vi "Starter Kit 2.0 Custom FPGA Main.vi"() -> ()   [LabVIEW 2011]
doc: "This VI implements the low level control of the motors and sensor for the Starter Kit 2.0 robot. The functionality of this VI is similar to the fixed FPGA personality used by the Starter Kit API."
uses:
  <vilib>/Platform/TimedLoop/XDataNode/timing_clust.ctl
  <vilib>/Platform/TimedLoop/XDataNode/nitl_modes.ctl
  <vilib>/Platform/TimedLoop/XDataNode/wakeup.ctl
  <vilib>/robotics/Utilities/Encoder Count Encoding.ctl
  Support VIs/Starter Kit 2.0 FPGA Globals.vi
  <vilib>/robotics/Utilities/FPGA Utilities/Count Two Phase Digital Encoder.vi
  <vilib>/rvi/eio/common/nirviEmuTemplateMethod_errors.vi
  <vilib>/robotics/Utilities/FPGA Utilities/Generate Digital Pulse (uSec).vi
  <vilib>/Platform/TimedLoop/XDataNode/XDataNode.xnode
  <vilib>/eio/EIONode/EIONode.xnode
  <vilib>/addons/control/pid/fpga.llb/XNode/niFpgaPID.xnode
  <vilib>/Platform/TimedLoop/XDataNode/XDNodeRunTimeDep.lvlib
  <vilib>/robotics/Utilities/NI_Robotics Utilities.lvlib
  <vilib>/robotics/Utilities/FPGA Utilities/NI_Robotics_FPGA Utilities.lvlib
  <instrlib>/Parallax PING)))/FPGA/NI_Robotics_Parallax PING))) (FPGA).lvlib
  <instrlib>/Hitec HS400 Series/FPGA/NI_Robotics_Hitec HS400 Series (FPGA).lvlib
  <instrlib>/Devantech CMPS03/FPGA/NI_Robotics_Devantech CMPS03 (FPGA).lvlib
panel:
  out "right counts":i32
  out "left counts":i32
  out "CMPS03 angle":fxp<+,20,16>
  out "CMPS 03 timed out":bool
  in  "FPGA LED":bool
  in  "ModB/AO0":fxp<+/-,20,5> format="%.17g"
  in  "ModB/AO1":fxp<+/-,20,5> format="%.17g"
  out "ModA/AI0":fxp<+/-,26,5> format="%.23g"
  out "ModA/AI1":fxp<+/-,26,5> format="%.23g"
  in  "Port7/DIO0_PWM":T1={"period (us)"=20000, "pulse width (us)"=1500}
  in  "Port7/DIO1_PWM":T1={"period (us)"=20000, "pulse width (us)"=1500}
  in  "Port3/DIO1":bool
  in  "Port3/DIO1_write":bool
  in  "Port3/DIO0":bool
  in  "Port3/DIO0_write":bool
  in  "hs400_0_ccw offset":fxp<+/-,32,4>
  in  "hs400_0_ccw angle":fxp<+/-,32,4>
  out "PING)))_0_timeout":bool
  out "PING)))_0_dist":fxp<+,32,8> format="%.27g"
  out "DCmotor_1_ccw vel":fxp<+/-,32,11>
  out "DCmotor_0_ccw vel":fxp<+/-,32,11>
  in  "DCmotor_1_ccw vel sp":fxp<+/-,32,11>
  in  "DCmotor_0_ccw vel sp":fxp<+/-,32,11>
  in  "stop":bool
  in  "motor PID gains":T2={"proportional gain (Kc)"=0.25, "integral gain (Kc*Ts/Ti)"=0.08984375, "derivative gain (Kc*Td/Ts)"=0.01171875}
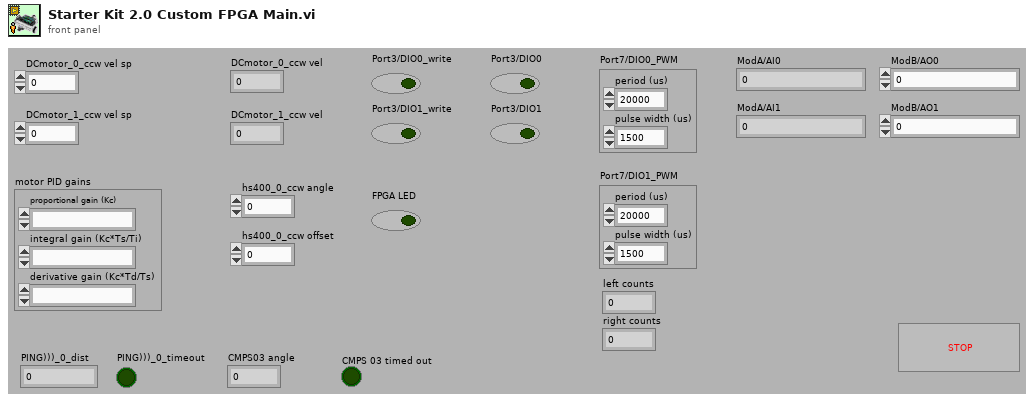
[diagram p1: front panel]
types:
  T1 = cluster{"period (us)":u32, "pulse width (us)":u32}
  T2 = cluster{"proportional gain (Kc)":fxp<+/-,16,8>, "integral gain (Kc*Ts/Ti)":fxp<+/-,16,8>, "derivative gain (Kc*Td/Ts)":fxp<+/-,16,8>}
  T3 = cluster{"PID gains":cluster{"proportional gain (Kc)":fxp<+/-,16,8>, "integral gain (Kc*Ts/Ti)":fxp<+/-,16,8>, "derivative gain (Kc*Td/Ts)":fxp<+/-,16,8>}, "output range":cluster{"output high":fxp<+/-,16,16>, "output low":fxp<+/-,16,16>}, "setpoint":fxp<+/-,16,16>, "channel index":u16}
  T4 = cluster{"PID gains (x 2^8)":cluster{"proportional gain (Kc)":i16, "integral gain (Kc*Ts/Ti)":i16, "derivative gain (Kc*Td/Ts)":i16}, "output range":cluster{"output high":i16, "output low":i16}, "setpoint":i16, "channel index":u16}
  T5 = typedef "XDNodeRunTimeDep.lvlib/timing_clust.ctl" = cluster{"Expected End [f-1]":u64, "Actual End [f-1]":u64, "Finished Late? [f-1]":bool, "Expected End [i-1]":u64, "Actual End [i-1]":u64, "Finished Late? [i-1]":bool, "Expected Start [i]":u64, "Actual Start [i]":u64, "Expected Start [f]":u64, "Actual Start [f]":u64, "Source Name":string, "Structure Name":string, "Period":i64, "Deadline":i64, "Offset":i64, "Start":i64, "Priority":i32, "Timeout":i32, "Mode":T6, "Wakeup Reason":T7, "Error":errorcluster, "Source Type":string, "Secondary Source Type":string, "Global End Time":u64, "Global Start Time":u64, "Frame Duration":u64, "Iteration Duration":u64, "Assigned CPU":i32, "I/O Scan Engine Mode":u32}
  T6 = typedef "XDNodeRunTimeDep.lvlib/nitl_modes.ctl" = enum32{"No Change", "Process missed periods, maintain original phase", "Discard missed periods, maintain original phase", "Process missed periods, ignore original phase", "Discard missed periods, ignore original phase"}
  T7 = typedef "XDNodeRunTimeDep.lvlib/wakeup.ctl" = enum32{"Normal", "Aborted", "Asynchronous wakeup", "Timing source error", "Timed loop error", "Timeout"}
  T8 = typedef "NI_Robotics Utilities.lvlib/Encoder Count Encoding.ctl" = enum16{"X1", "X2", "X4"}
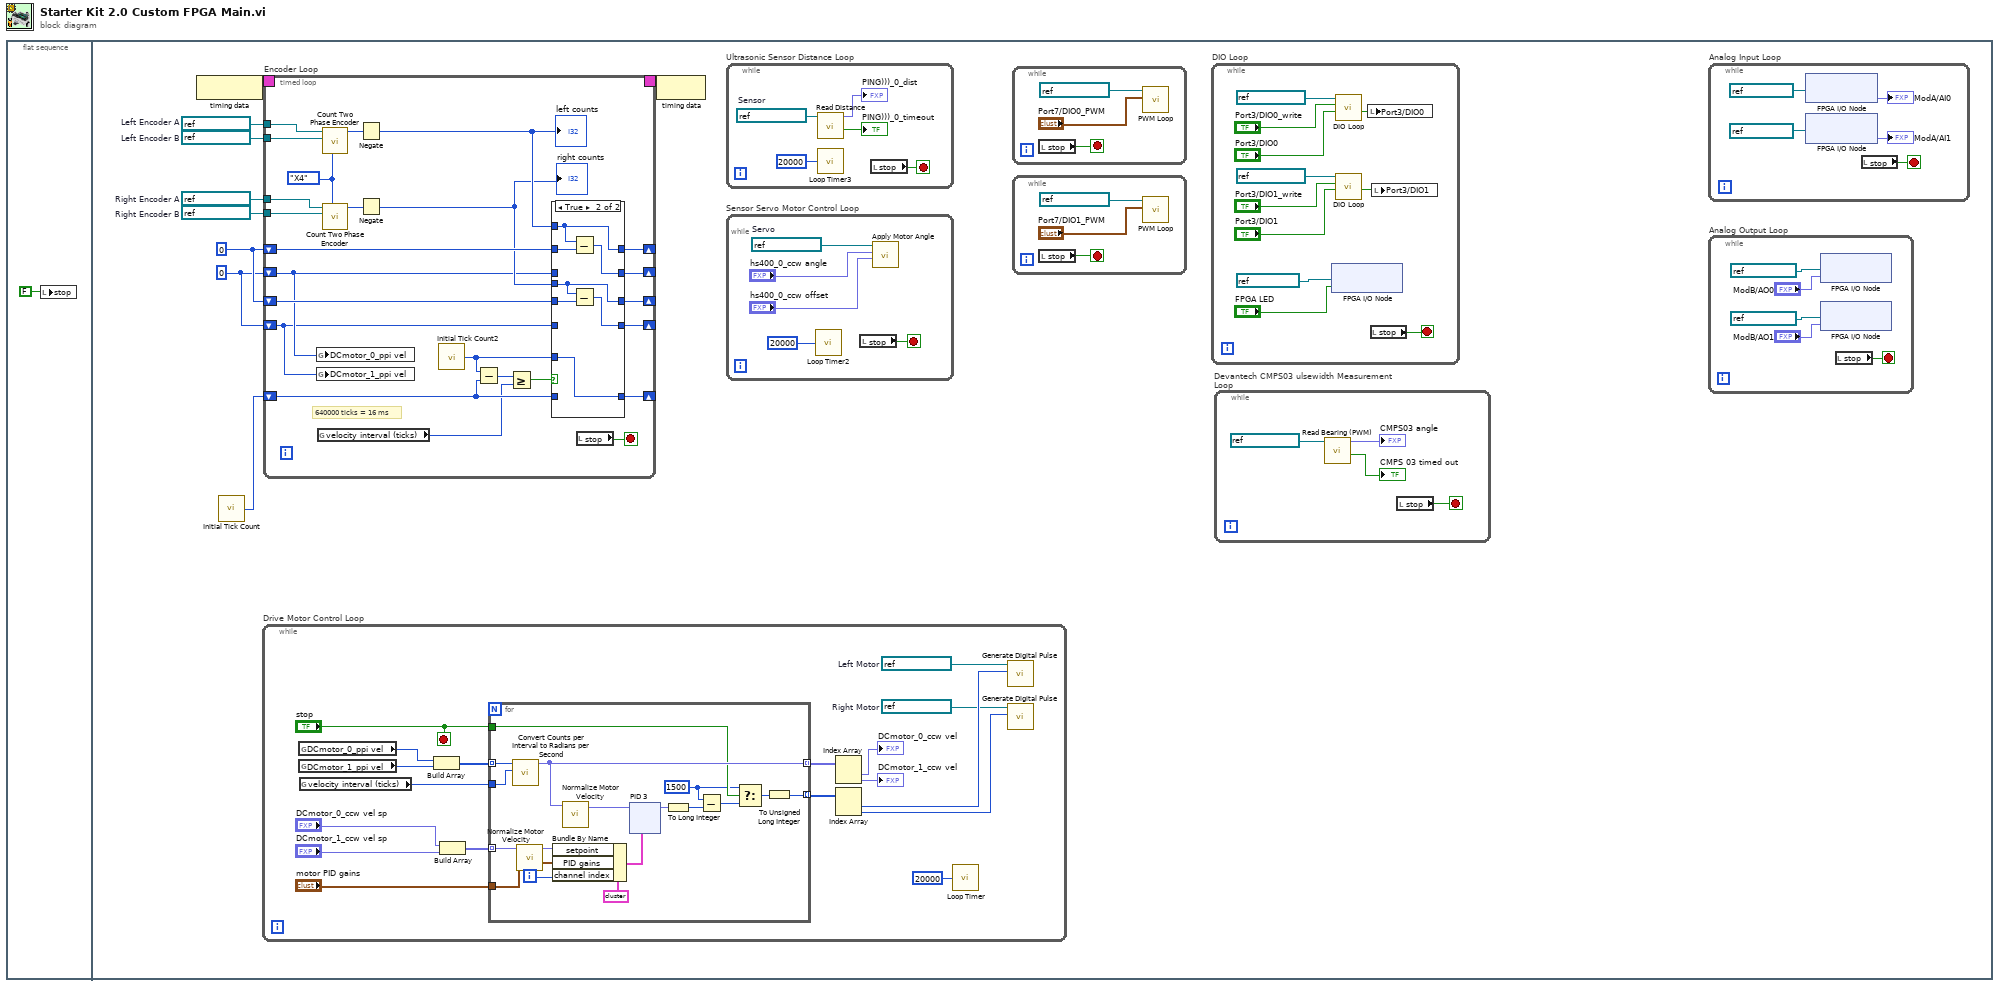
[diagram p0: block diagram]
diagram:
  n1 = flat-sequence {
    frame #0 {
      n2 = local write "stop"(FALSE ("stop")) -> ()
    }
    frame #1 {
      w2 = refnum<k21> "Port0/DIO3"  # Right Encoder B
      w3 = refnum<k21> "Port0/DIO2"  # Right Encoder A
      w4 = refnum<k21> "Port0/DIO1"  # Left Encoder B
      w5 = refnum<k21> "Port0/DIO0"  # Left Encoder A
      w6 = 0
      w7 = 0 ("Reset Position Value")
      n3 = node-c288() -> (w10:T5)
      n4 = call "Initial Tick Count"() -> ("Tick Count(Ticks)"=w8:u32)
      n5 = while "Drive Motor Control Loop" {
        stop <- "stop" stop-if-true
        w48 = refnum<k21> "Port0/DIO5"  # Right Motor
        w49 = refnum<k21> "Port0/DIO4"  # Left Motor
        n6 = global read "Starter Kit 2.0 FPGA Globals.vi" "DCmotor_0_ppi vel"() -> (w43:i32)
        n7 = global read "Starter Kit 2.0 FPGA Globals.vi" "DCmotor_1_ppi vel"() -> (w42:i32)
        n8 = global read "Starter Kit 2.0 FPGA Globals.vi" "velocity interval (ticks)"() -> (w44:u32)
        n9 = Build Array(w43, w42) -> (w57:i32[])
        n10 = Build Array("DCmotor_0_ccw vel sp", "DCmotor_1_ccw vel sp") -> (w55:fxp<+/-,32,11>[])
        n11 = for {
          tunnel: "motor PID gains" -> [w73]
          tunnel: w57 -> [w72] mode=indexing
          tunnel: w44 -> [w71]
          tunnel: [w70] -> w56 mode=indexing
          tunnel: w55 -> [w60] mode=indexing
          tunnel: "stop" -> [w64]
          tunnel: [w66] -> w54 mode=indexing
          i -> [w74]
          w63 = 1500 ("y")
          n12 = call "Convert Counts per Interval to Radians per Second.vi"("interval (ticks)"=w71, "velocity (pulses/interval)"=w72) -> ("velocity (rad/s)"=w70:fxp<+/-,32,11>)  [unwired: 9 in]
          n13 = call "Normalize Motor Velocity.vi"("velocity (rad/s)"=w60) -> ("normalized velocity"=w67:fxp<+/-,16,16>)  [unwired: 10 in]
          n14 = Bundle By Name(cluster=T3 {"PID gains"={"proportional gain (Kc)"=0.00390625, "integral gain (Kc*Ts/Ti)"=0.00390625, "derivative gain (Kc*Td/Ts)"=0.00390625}, "output range"={"output high"=500.0, "output low"=-500.0}, "setpoint"=0.0, "channel index"=0} ("configuration"), "setpoint"=w67, "PID gains"=w73, "channel index"=w74) -> (w75:T3)
          n15 = call "Normalize Motor Velocity.vi"("velocity (rad/s)"=w70) -> ("normalized velocity"=w69:fxp<+/-,16,16>)  [unwired: 10 in]
          n16 = xnode ("PID 3")("process variable"=w69, "configuration"=w75) -> ("output"=w68:fxp<+/-,16,16>)  [unwired: 1 in, 1 out]
          n17 = To Long Integer(number=w68) -> (32bit integer=w65:i32)
          n18 = Subtract(x=w63, y=w65) -> (x-y=w62:i32)
          n19 = Select(t=w63, s=w64, f=w62) -> (s? t:f=w61:i32)
          n20 = To Unsigned Long Integer(number=w61) -> (unsigned 32bit integer=w66:u32)
        }
        n21 = Index Array(array=w56) -> (element #1=→"DCmotor_0_ccw vel":fxp<+/-,32,11>, element #2=→"DCmotor_1_ccw vel":fxp<+/-,32,11>)  [unwired: 2 in]
        n22 = Index Array(array=w54) -> (element #1=w53:u32, element #2=w50:u32)  [unwired: 2 in]
        n23 = call "Loop Timer"("Count(uSec)"=u32 20000) -> ()  [unwired: 1 out]
        n24 = call-poly <vilib>:"Generate Digital Pulse.vi"("pulse width (uSec)"=w53, "FPGA digital output"=w49) -> ()  [unwired: 10 in]
        n25 = call-poly <vilib>:"Generate Digital Pulse.vi"("pulse width (uSec)"=w50, "FPGA digital output"=w48) -> ()  [unwired: 10 in]
      }
      n26 = timed-loop "Encoder Loop" {
        timing: w10 -> [_]
        timing-out: [_] -> w9
        shift-right: [w130] -> _
        shift-left: w8 -> [w135]
        shift-right: [w131] -> _
        shift-left: w7 -> [w133]
        shift-right: [w132] -> _
        shift-left: w6 -> [w116]
        shift-right: [w128] -> _
        shift-left: w7 -> [w129]
        shift-right: [w127] -> _
        shift-left: w6 -> [w115]
        tunnel: w5 -> [w123]
        tunnel: w4 -> [w122]
        tunnel: w3 -> [w120]
        tunnel: w2 -> [w119]
        stop <- w124 stop-if-true
        w117 = Encoder_Count_Encoding."X4" ("count multiplier (X1)")
        # "640000 ticks = 16 ms"
        n27 = global write "Starter Kit 2.0 FPGA Globals.vi" "DCmotor_0_ppi vel"(w116) -> ()
        n28 = global write "Starter Kit 2.0 FPGA Globals.vi" "DCmotor_1_ppi vel"(w115) -> ()
        n29 = global read "Starter Kit 2.0 FPGA Globals.vi" "velocity interval (ticks)"() -> (w114:u32)
        n30 = call-poly <vilib>:"Count Two Phase Encoder.vi"("count encoding (X1)"=w117, "phase B FPGA digital input"=w122, "phase A FPGA digital input"=w123) -> ("new count"=w121:i32)  [unwired: 7 in, 1 out]
        n31 = call-poly <vilib>:"Count Two Phase Encoder.vi"("count encoding (X1)"=w117, "phase B FPGA digital input"=w119, "phase A FPGA digital input"=w120) -> ("new count"=w118:i32)  [unwired: 7 in, 1 out]
        n32 = Negate(x=w121) -> (-x=w126:i32)
        "left counts" <- w126
        n33 = Negate(x=w118) -> (-x=w125:i32)
        "right counts" <- w125
        n34 = call "Initial Tick Count2"() -> ("Tick Count(Ticks)"=w134:u32)
        n35 = Subtract(x=w134, y=w135) -> (x-y=w137:u32)
        n36 = Greater Or Equal?(x=w137, y=w114) -> (x >= y?=w136:bool)
        n37 = case shown="True" w136 {
          tunnel: w134 -> [_ w148]
          tunnel: w135 -> [w142 _]
          tunnel: [w142 w148] -> w130
          tunnel: w133 -> [w141 w149]
          tunnel: [w141 w147] -> w131
          tunnel: w126 -> [_ w147]
          tunnel: [w140 w146] -> w132
          tunnel: w116 -> [w140 _]
          tunnel: w129 -> [w139 w145]
          tunnel: w115 -> [w138 _]
          tunnel: [w139 w144] -> w128
          tunnel: [w138 w143] -> w127
          tunnel: w125 -> [_ w144]
          frame False {
          }
          frame True {
            n38 = Subtract(x=w147, y=w149) -> (x-y=w146:i32)
            n39 = Subtract(x=w144, y=w145) -> (x-y=w143:i32)
          }
        }
        n40 = local read "stop"() -> (w124:bool)
      }
      n41 = node-c288(w9) -> ()
      n42 = while "Ultrasonic Sensor Distance Loop" {
        stop <- w112 stop-if-true
        w109 = refnum<k21> "Port0/DIO6"  # Sensor
        n43 = call <instrlib>:"Read Distance.vi"("trigger/echo line"=w109) -> ("timed out?"=→"PING)))_0_timeout":bool, "distance (m)"=→"PING)))_0_dist":fxp<+,32,8>)  [unwired: 9 in]
        n44 = call "Loop Timer3"("Count(uSec)"=u32 20000 ("sensor period (15000 us)")) -> ()  [unwired: 1 out]
        n45 = local read "stop"() -> (w112:bool)
      }
      n46 = while "Sensor Servo Motor Control Loop" {
        stop <- w108 stop-if-true
        w107 = refnum<k21> "Port0/DIO7"  # Servo
        n47 = call "Loop Timer2"("Count(uSec)"=u32 20000) -> ()  [unwired: 1 out]
        n48 = local read "stop"() -> (w108:bool)
        n49 = call <instrlib>:"Apply Motor Angle.vi"("ccw angle offset (rad)"="hs400_0_ccw offset", "ccw angle (rad)"="hs400_0_ccw angle", "digital output line"=w107) -> ()  [unwired: 9 in]
      }
      n50 = while {
        stop <- w41 stop-if-true
        n51 = local read "stop"() -> (w41:bool)
        n52 = call "PWM Loop.vi"("PWM"="Port7/DIO0_PWM", "FPGA I/O"=refnum<k21> "Port7/DIO0" ("FPGA I/O In")) -> ()  [unwired: 10 in]
      }
      n53 = while {
        stop <- w38 stop-if-true
        n54 = local read "stop"() -> (w38:bool)
        n55 = call "PWM Loop.vi"("PWM"="Port7/DIO1_PWM", "FPGA I/O"=refnum<k21> "Port7/DIO1" ("FPGA I/O In")) -> ()  [unwired: 10 in]
      }
      n56 = while "DIO Loop" {
        stop <- w27 stop-if-true
        n57 = xnode "FPGA I/O Node"("I/O Item"="FPGA LED", "FPGA I/O In"=refnum<k21> "FPGA LED" ("LED")) -> ()  [unwired: 1 out]
        n58 = call "DIO Loop.vi"("DIO value in"="Port3/DIO0", "enable output"="Port3/DIO0_write", "DIO line"=refnum<k21> "Port3/DIO0" ("FPGA I/O")) -> ("DIO value out"=w32:bool)  [unwired: 8 in]
        n59 = call "DIO Loop.vi"("DIO value in"="Port3/DIO1", "enable output"="Port3/DIO1_write", "DIO line"=refnum<k21> "Port3/DIO1" ("FPGA I/O")) -> ("DIO value out"=w31:bool)  [unwired: 8 in]
        n60 = local write "Port3/DIO0"(w32) -> ()
        n61 = local read "stop"() -> (w27:bool)
        n62 = local write "Port3/DIO1"(w31) -> ()
      }
      n63 = while "Devantech CMPS03 ulsewidth Measurement Loop" {
        stop <- w11 stop-if-true
        n64 = call <instrlib>:"Read Bearing (PWM).vi"("PWM line"=refnum<k21> "Port4/DIO6" ("FPGA I/O In")) -> ("timed out"=→"CMPS 03 timed out":bool, "bearing (degree)"=→"CMPS03 angle":fxp<+,20,16>)  [unwired: 9 in]
        n65 = local read "stop"() -> (w11:bool)
      }
      n66 = while "Analog Input Loop" {
        stop <- w24 stop-if-true
        n67 = xnode "FPGA I/O Node"("FPGA I/O In"=refnum<k21> "ModA/AI0") -> ("I/O Item"=→"ModA/AI0":fxp<+/-,26,5>)  [unwired: 1 out]
        n68 = xnode "FPGA I/O Node"("FPGA I/O In"=refnum<k21> "ModA/AI1") -> ("I/O Item"=→"ModA/AI1":fxp<+/-,26,5>)  [unwired: 1 out]
        n69 = local read "stop"() -> (w24:bool)
      }
      n70 = while "Analog Output Loop" {
        stop <- w18 stop-if-true
        n71 = xnode "FPGA I/O Node"("I/O Item"="ModB/AO0", "FPGA I/O In"=refnum<k21> "ModB/AO0") -> ()  [unwired: 1 out]
        n72 = xnode "FPGA I/O Node"("I/O Item"="ModB/AO1", "FPGA I/O In"=refnum<k21> "ModB/AO1") -> ()  [unwired: 1 out]
        n73 = local read "stop"() -> (w18:bool)
      }
    }
  }
